vi "alignTopWith.vi"(6 "useControlBodyOnly":bool, 8 "error in (no error)":errorcluster, 10 "anchorObject":refnum<vi>, 11 "movingObject":refnum<vi>) -> (0 "error out":errorcluster, 2 "anchorObject(dup)":refnum<vi>, 3 "movingObject(dup)":refnum<vi>)   [LabVIEW 2023]
doc: "Align top the 'movingObject' with the 'anchorObject'.\n\nOnly the Y position of the item is modified.\nThe X position is preserved"
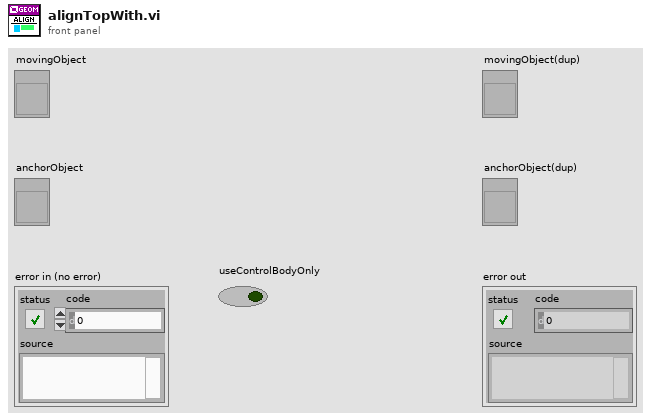
[diagram p1: front panel]
types:
  T1 = cluster{"left":i32, "top":i32, "right":i32, "bottom":i32}
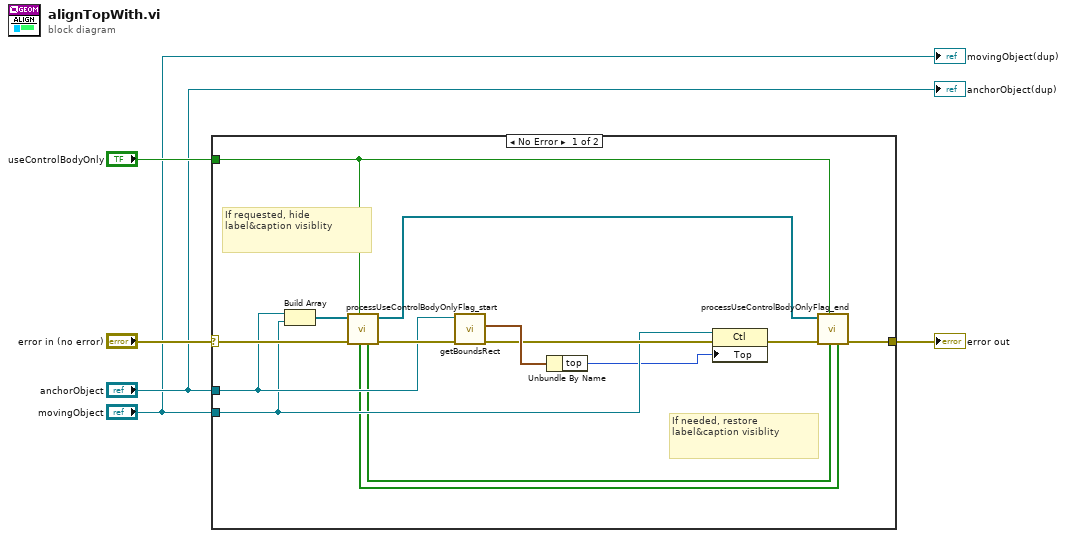
[diagram p0: block diagram]
diagram:
  n1 = case shown="No Error" "error in (no error)" {
    selector: "error in (no error)" -> [w19 w20]
    tunnel: [w16 w20] -> w5
    tunnel: "anchorObject" -> [w14 _]
    tunnel: "useControlBodyOnly" -> [w9 _]
    tunnel: "movingObject" -> [w11 _]
    frame No Error {
      # "If needed, restore label&caption visiblity"
      # "If requested, hide label&caption visiblity"
      n2 = Build Array(w14, w11) -> (w18:refnum<vi>[])
      n3 = call "processUseControlBodyOnlyFlag_start.vi"("useControlBodyOnly"=w9, "error in (no error)"=w19, "refList"=w18) -> ("error out"=w15:errorcluster, "refList(dup)"=w17:refnum<vi>[], "LabelVisibilityList"=w8:bool[], "captionVisibilityList"=w7:bool[])  [unwired: 5 in]
      n4 = call "getBoundsRect.vi"("error in (no error)"=w15, "ref"=w14) -> ("error out"=w12:errorcluster, "rect"=w13:T1)  [unwired: 7 in, 1 out]
      n5 = Unbundle By Name(w13) -> ("top"=w6:i32)
      n6 = property class="Ctl"(reference=w11, error in=w12, "Top"=w6) -> (error out=w10:errorcluster)  [unwired: 1 out]
      n7 = call "processUseControlBodyOnlyFlag_end.vi"("captionVisibilityList"=w7, "LabelVisibilityList"=w8, "useControlBodyOnly"=w9, "error in (no error)"=w10, "refList"=w17) -> ("error out"=w16:errorcluster)  [unwired: 5 in, 1 out]
    }
    frame Error {
    }
  }
  "error out" <- w5
  "movingObject(dup)" <- "movingObject"
  "anchorObject(dup)" <- "anchorObject"
